vi "Binary Formula Decoding.vi"(8 "Error In":errorcluster, 10 "Variables":string[](array[string]), 11 "Formula":string) -> (0 "Error Out":errorcluster, 3 "Array of Binary Operation Steps":T1[](array[typedef]))   [LabVIEW 2021, in "Formula.lvlib"]
uses:
  Formula.lvlib
  Binary Formula Step.ctl
  Binary Operator.ctl
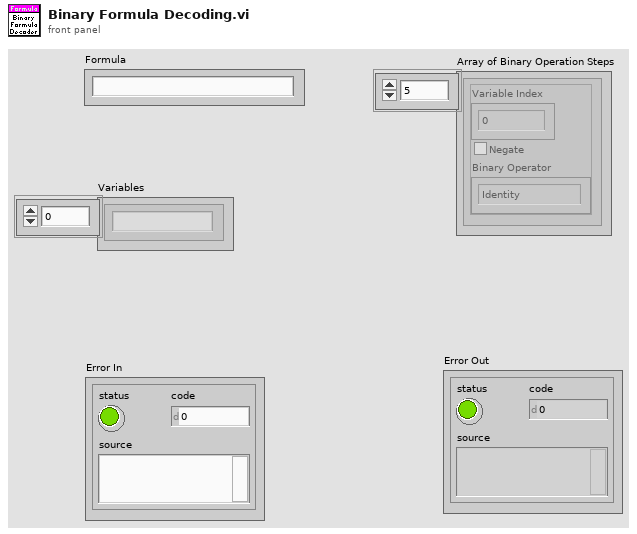
[diagram p1: front panel]
types:
  T1 = typedef "Formula.lvlib/Binary Formula Step.ctl" = cluster{"Variable Index":i32, "Negate":bool, "Binary Operator":T2}
  T2 = typedef "Formula.lvlib/Binary Operator.ctl" = enum16{"Identity", "AND", "OR"}
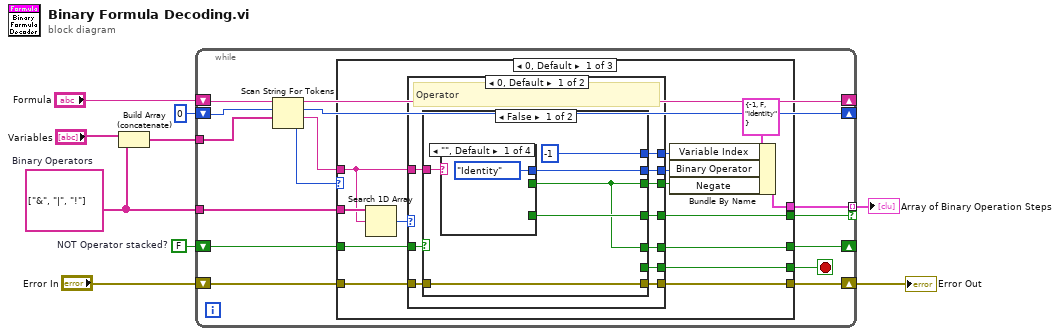
[diagram p0: block diagram]
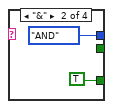
[diagram p2: hidden frame]
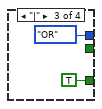
[diagram p3: hidden frame]
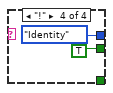
[diagram p4: hidden frame]
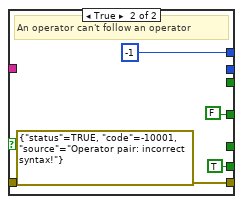
[diagram p5: hidden frame]
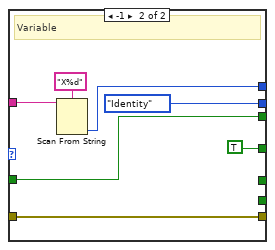
[diagram p6: hidden frame]
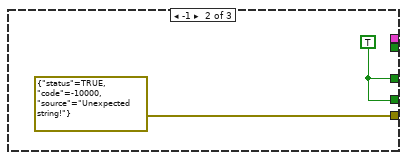
[diagram p7: hidden frame]
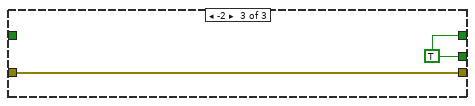
[diagram p8: hidden frame]
diagram:
  w4 = FALSE  # NOT Operator stacked?
  w5 = string[] ["&", "|", "!"]  # Binary Operators
  n1 = Build Array (concatenate)("Variables", w5) -> (w7:string[])
  n2 = while {
    shift-right: [w23] -> _
    shift-left: "Formula" -> [w24]
    tunnel: w7 -> [w22]
    shift-right: [w20] -> _
    shift-left: 0 ("offset past token") -> [w21]
    tunnel: w5 -> [w16]
    shift-right: [w14] -> _
    shift-left: w4 -> [w13]
    tunnel: [w15] -> w3 mode=indexing if=w12
    shift-right: [w10] -> w1
    shift-left: "Error In" -> [w11]
    stop <- w17 stop-if-true
    n3 = Scan String For Tokens(7:w22, 8:w21, 9:w24) -> (0:w19:i32, 1:w18:string, 2:w20:i32, 3:w23:string)  [unwired: 3 in]
    n4 = case shown="0, Default" w19 {
      tunnel: w18 -> [w36 _ _]
      tunnel: [w28 w74 w76] -> w17
      tunnel: w16 -> [w38 _ _]
      tunnel: [w25 w74 w76] -> w14
      tunnel: [w33 _ _] -> w15
      tunnel: w13 -> [w32 _ _]
      tunnel: [w29 _ _] -> w12
      tunnel: w11 -> [w26 _ w75]
      tunnel: [w27 errorcluster {"status"=TRUE, "code"=-10000, "source"="Unexpected string!"} ("Error Out") w75] -> w10
      frame 0, Default {
        n5 = Search 1D Array(1D array=w38, element=w36) -> (index of element=w37:i32)  [unwired: 1 in]
        n6 = case shown="0, Default" w37 {
          tunnel: w36 -> [w48 w72]
          tunnel: [w47 Binary_Operator."Identity" ("Binary Operator")] -> w35
          tunnel: [w45 w69] -> w30
          tunnel: w32 -> [w43 w69]
          tunnel: [w46 w68] -> w31
          tunnel: [w44 TRUE] -> w29
          tunnel: [w42 _] -> w28
          tunnel: [w41 w66] -> w27
          tunnel: w26 -> [w40 w66]
          tunnel: [w39 _] -> w25
          frame 0, Default {
            # "Operator"
            n7 = case shown="False" w43 {
              tunnel: w48 -> [w54 _]
              tunnel: [w53 _] -> w47
              tunnel: [-1 -1] -> w46
              tunnel: [w49 _] -> w45
              tunnel: [w51 FALSE] -> w44
              tunnel: [_ TRUE] -> w42
              tunnel: [w50 errorcluster {"status"=TRUE, "code"=-10001, "source"="Operator pair: incorrect syntax!"} ("Error In")] -> w41
              tunnel: w40 -> [w50 _]
              tunnel: [w49 _] -> w39
              frame False {
                n8 = case shown="\"\", Default" w54 {
                  tunnel: [Binary_Operator."Identity" ("Binary Operator") Binary_Operator."AND" ("Binary Operator") Binary_Operator."OR" ("Binary Operator") Binary_Operator."Identity" ("Binary Operator")] -> w53
                  tunnel: [_ _ _ TRUE ("Negate")] -> w49
                  tunnel: [_ TRUE TRUE _] -> w51
                  frame "", Default {
                  }
                  frame "&" {
                  }
                  frame "|" {
                  }
                  frame "!" {
                  }
                }
              }
              frame True {
                # "An operator can't follow an operator"
              }
            }
          }
          frame -1 {
            # "Variable"
            n9 = Scan From String(format string="X%d", input string=w72) -> (output 1=w68:i32)  [unwired: 3 in, 3 out]
          }
        }
        n10 = Bundle By Name(cluster=T1 {"Variable Index"=-1, "Negate"=FALSE, "Binary Operator"=enum."Identity"} ("Binary Operation Step"), "Variable Index"=w31, "Binary Operator"=w35, "Negate"=w30) -> (w33:T1)
      }
      frame -1 {
        w74 = TRUE
      }
      frame -2 {
        w76 = TRUE
      }
    }
  }
  "Array of Binary Operation Steps" <- w3
  "Error Out" <- w1
